vi "CreateSystemEventStream.vi"() -> (2 "Event Stream Out":refnum<user-event>, 3 "Event Registration Refnum out":refnum<event-registration>)   [LabVIEW 2017]
uses:
  Types/SystemEventDataStruct.ctl
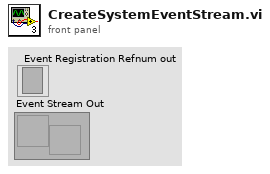
[diagram p1: front panel]
types:
  T1 = typedef "SystemEventDataStruct.ctl" = cluster{"Data":variant, "name":string}
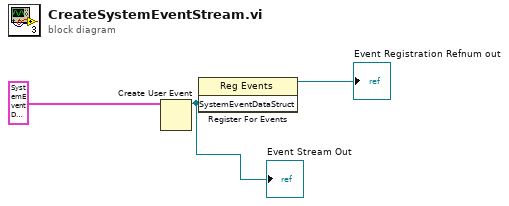
[diagram p0: block diagram]
diagram:
  n1 = Create User Event(user event datatype=T1 {"Data"=variant, "name"=""} ("SystemEventDataStruct")) -> (user event=w3:refnum<user-event>)  [unwired: 1 in, 1 out]
  "Event Stream Out" <- w3
  n2 = register-events(w3) -> (reference out=→"Event Registration Refnum out":refnum<event-registration>)  [unwired: 2 in, 1 out]
